vi "Make shift signal.vi"(6 "cyclesperstim":dbl=20.0, 7 "Output freq (Hz)":dbl=50.0, 9 "sinfreq":dbl=1.5 caption="sinefreq", 10 "total time":dbl=20.0, 11 "pulse data":T3) -> (3 "sine signal":dbl[](array[numeric]))   [LabVIEW 2013]
uses:
  Pulse data.ctl
  Phases.ctl
  <vilib>/Analysis/1siggen.llb/Ramp Pattern by Delta.vi
  <vilib>/gmath/NI_Gmath.lvlib
  <vilib>/Analysis/NI_AALBase.lvlib
panel:
  out "XY Graph":T1(graph)
  out "phases":T2
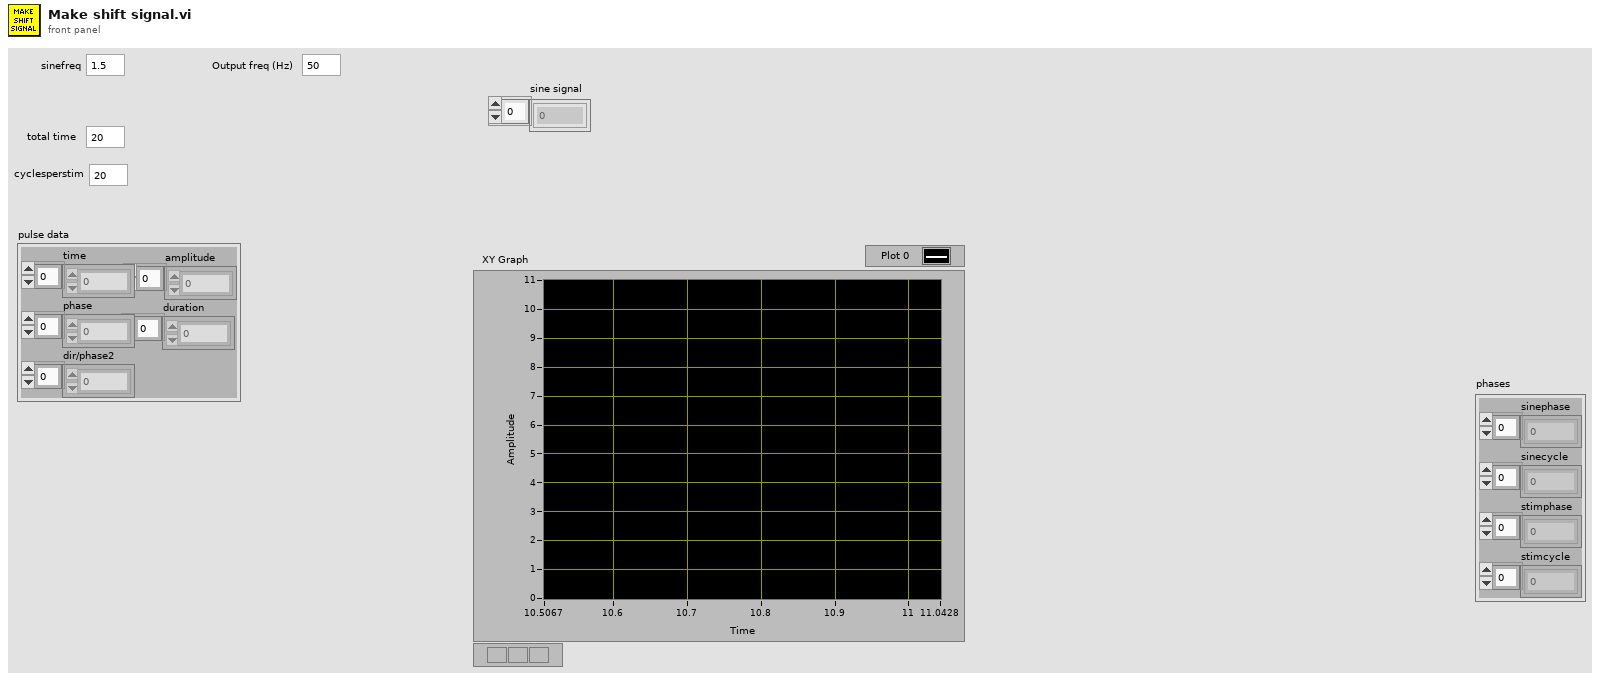
[diagram p1: front panel]
types:
  T1 = cluster{"ramp signal":dbl[], "Ramp Pattern":dbl[]}
  T2 = typedef "Phases.ctl" = cluster{"sinephase":dbl[], "sinecycle":dbl[], "stimphase":dbl[], "stimcycle":dbl[]}
  T3 = typedef "Pulse data.ctl" = cluster{"time":dbl[], "phase":dbl[], "dir/phase2":dbl[], "amplitude":dbl[], "duration":dbl[]}
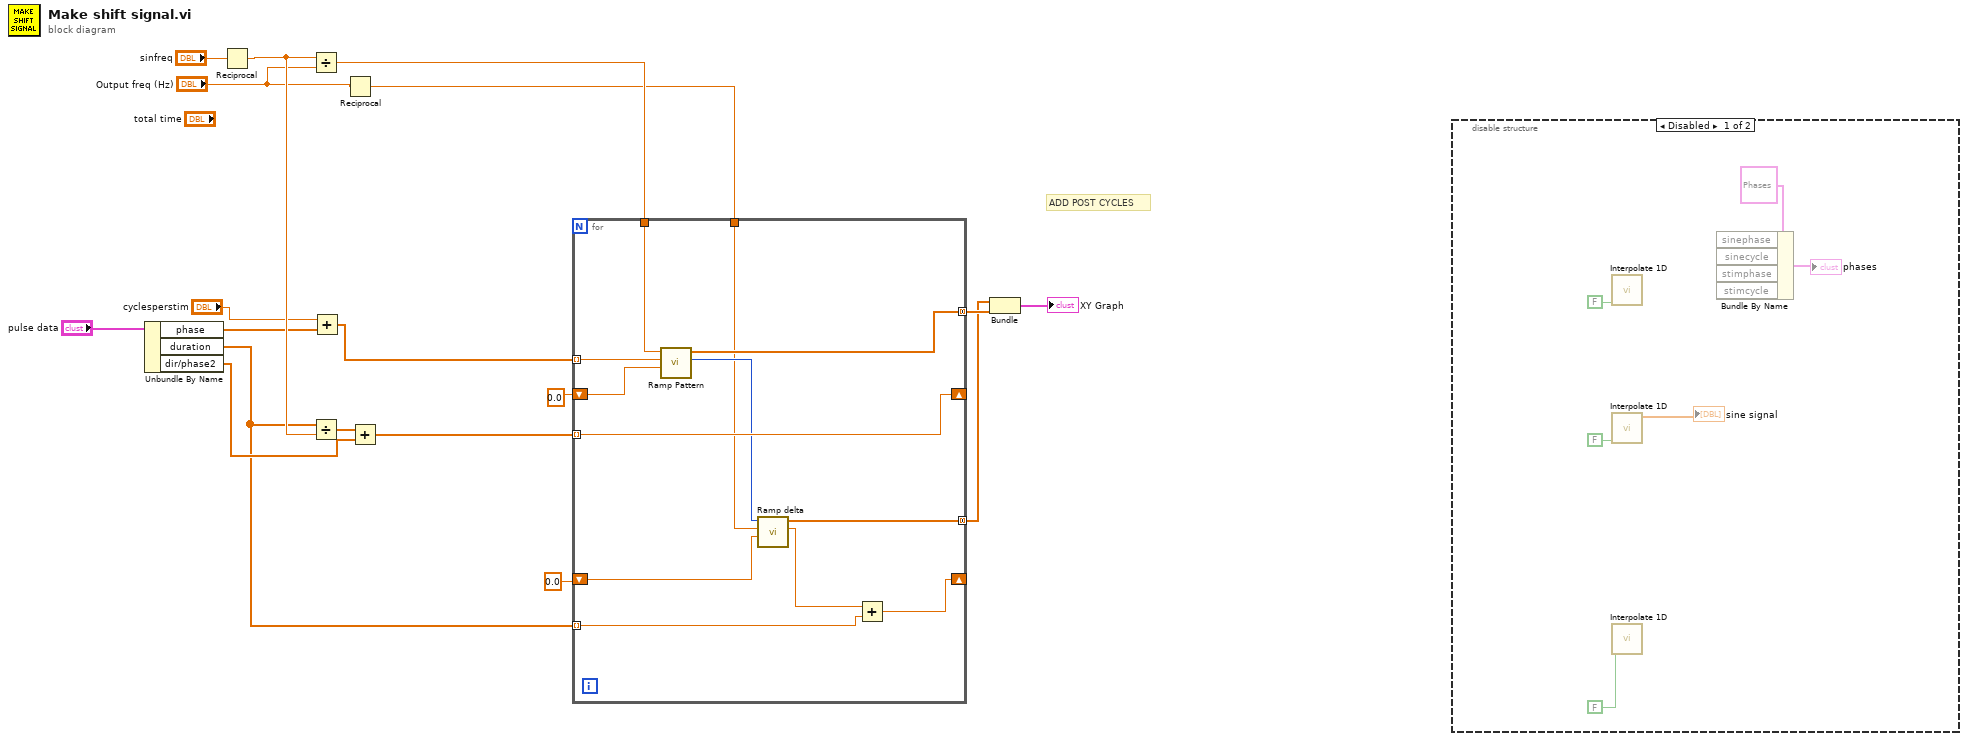
[diagram p0: block diagram]
diagram:
  # "ADD POST CYCLES"
  n1 = Unbundle By Name("pulse data") -> ("phase"=w11:dbl[], "duration"=w1:dbl[], "dir/phase2"=w13:dbl[])
  n2 = Reciprocal(x="sinfreq") -> (1/x=w15:dbl)
  n3 = Divide(x=w15, y="Output freq (Hz)") -> (x/y=w7:dbl)
  n4 = Divide(x=w1, y=w15) -> (x/y=w14:dbl[])
  n5 = Add(x="cyclesperstim", y=w11) -> (x+y=w9:dbl[])
  n6 = Reciprocal(x="Output freq (Hz)") -> (1/x=w5:dbl)
  n7 = Add(x=w14, y=w13) -> (x+y=w12:dbl[])
  n8 = for {
    shift-right: [w30] -> _
    shift-left: 0.0 ("element") -> [w29]
    tunnel: w7 -> [w27]
    tunnel: w12 -> [w30] mode=indexing
    tunnel: w1 -> [w22] mode=indexing
    tunnel: w9 -> [w28] mode=indexing
    tunnel: [w26] -> w4 mode=concatenating
    shift-right: [w20] -> _
    shift-left: 0.0 ("element") -> [w23]
    tunnel: w5 -> [w24]
    tunnel: [w19] -> w3 mode=concatenating
    n9 = call-poly <vilib>:"Ramp Pattern.vi"("start"=w29, "end"=w28, "delta"=w27) -> ("samples"=w25:i32, "Ramp Pattern"=w26:dbl[])  [unwired: 6 in, 1 out]
    n10 = call "Ramp delta.vi"("start"=w23, "delta"=w24, "samples"=w25) -> ("last value"=w21:dbl, "ramp signal"=w19:dbl[])  [unwired: 7 in]
    n11 = Add(x=w21, y=w22) -> (x+y=w20:dbl)
  }
  n12 = Bundle("ramp signal"=w3, "Ramp Pattern"=w4) -> (→"XY Graph":T1)  [unwired: 1 in]
  n13 = disable-structure shown="Disabled" {
    frame Disabled {
      n14 = call <vilib>:"Interpolate 1D.vi"("X is monotonic"=FALSE) -> ()  [unwired: 8 in, 3 out]
      n15 = call <vilib>:"Interpolate 1D.vi"("X is monotonic"=FALSE) -> ("yi"=→"sine signal":dbl[])  [unwired: 8 in, 2 out]
      n16 = call <vilib>:"Interpolate 1D.vi"("X is monotonic"=FALSE) -> ()  [unwired: 8 in, 3 out]
      n17 = Bundle By Name(cluster=T2 {"sinephase"=array[5367 elements], "sinecycle"=array[5367 elements], "stimphase"=array[5367 elements], "stimcycle"=array[5367 elements]} ("phases")) -> (→"phases":T2)  [unwired: 4 in]
    }
    frame Enabled {
    }
  }
